vi "Read Configuration.vi"(8 "error in":errorcluster, 11 "Ballard MIL-STD 1553 custom device in":T1 format="%.0x") -> (0 "error out":errorcluster, 2 "1553 channels":T2[](array[typedef]), 3 "Ballard MIL-STD 1553 custom device out":T1 format="%.0x")   [LabVIEW 2020, in "Ballard MIL-STD-1553 Scripting.lvlib"]
uses:
  Ballard MIL-STD-1553 Scripting.lvlib
  <vilib>/NI VeriStand/Custom Device API/Custom Device Item Ref.ctl
  Shared/1553 Channel.ctl
  Shared/Address.ctl
  Shared/Message Definition.ctl
  Shared/Message Type.ctl
  Shared/Terminal Endpoint.ctl
  Shared/Parameter Definition.ctl
  <vilib>/NI VeriStand/Custom Device API/Custom Device API.lvlib
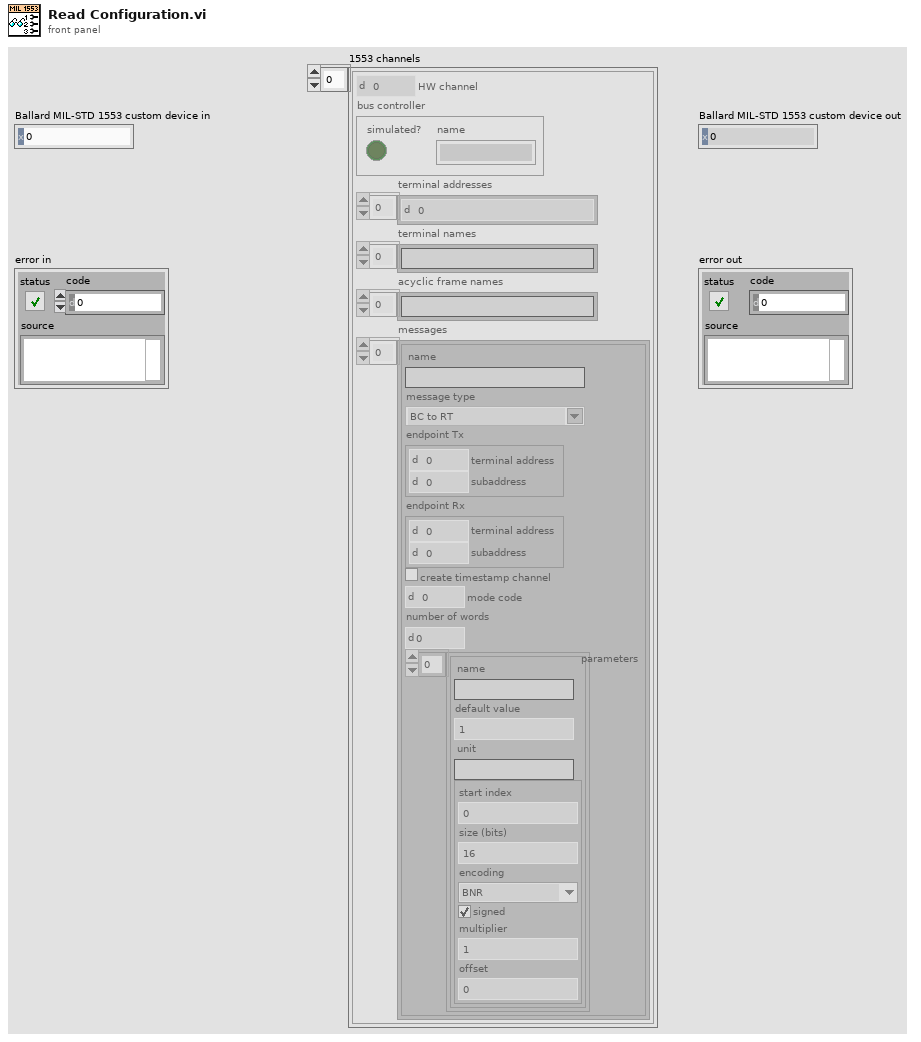
[diagram p1: front panel]
types:
  T1 = typedef "Custom Device API.lvlib/Custom Device Item Ref.ctl" = u64
  T2 = typedef "1553 Channel.ctl" = cluster{"HW channel":u16, "bus controller":cluster{"simulated?":bool, "name":string}, "terminal addresses":T3[], "terminal names":string[], "acyclic frame names":string[], "messages":T4[]}
  T3 = typedef "Address.ctl" = u16
  T4 = typedef "Message Definition.ctl" = cluster{"name":string, "message type":T5, "endpoint Tx":T6, "endpoint Rx":T6, "create timestamp channel":bool, "mode code":u16, "number of words":u16, "parameters":cluster{"name":string, "default value":dbl, "unit":string, "parameter definition":T7}[]}
  T5 = typedef "Message Type.ctl" = string
  T6 = typedef "Terminal Endpoint.ctl" = cluster{"terminal address":T3, "subaddress":T3}
  T7 = typedef "Parameter Definition.ctl" = cluster{"start index":i32, "size (bits)":i32, "encoding":enum16{"BNR", "BCD", "Discrete"}, "signed":bool, "multiplier":dbl, "offset":dbl}
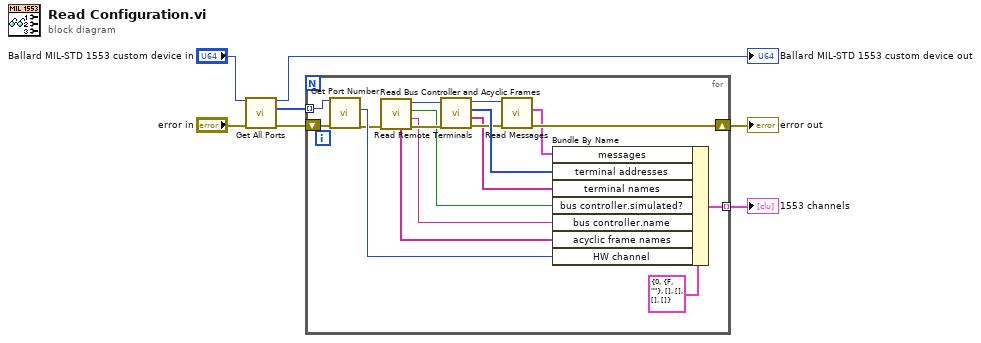
[diagram p0: block diagram]
diagram:
  n1 = call "Get All Ports.vi"("error in"="error in", "Ballard MIL-STD 1553 custom device in"="Ballard MIL-STD 1553 custom device in") -> ("error out"=w4:errorcluster, "ports"=w3:T1[], "Ballard MIL-STD 1553 custom device out"=→"Ballard MIL-STD 1553 custom device out":T1)  [unwired: 7 in]
  n2 = for {
    shift-right: [w16] -> w7
    shift-left: w4 -> [w24]
    tunnel: w3 -> [w23] mode=indexing
    tunnel: [w20] -> w1 mode=indexing
    n3 = call "Get Port Number.vi"("error in"=w24, "port in"=w23) -> ("error out"=w12:errorcluster, "port number"=w21:u16)  [unwired: 6 in, 2 out]
    n4 = call "Read Bus Controller and Acyclic Frames.vi"("error in"=w12) -> ("error out"=w13:errorcluster, "bus controller name"=w9:string, "bus controller found"=w10:bool, "port out"=w8:T1, "acyclic frame names"=w11:string[])  [unwired: 6 in]
    n5 = call "Read Remote Terminals.vi"("error in"=w13, "port in"=w8) -> ("error out"=w17:errorcluster, "terminal names"=w14:string[], "terminals"=w19:T3[], "port out"=w18:T1)  [unwired: 6 in]
    n6 = call "Read Messages.vi"("error in"=w17, "port in"=w18) -> ("error out"=w16:errorcluster, "messages"=w15:T4[])  [unwired: 7 in, 1 out]
    n7 = Bundle By Name(cluster=T2 {"HW channel"=0, "bus controller"={"simulated?"=FALSE, "name"=""}, "terminal addresses"=[], "terminal names"=[], "acyclic frame names"=[], "messages"=[]} ("1553 channel"), "messages"=w15, "terminal addresses"=w19, "terminal names"=w14, "bus controller.simulated?"=w10, "bus controller.name"=w9, "acyclic frame names"=w11, "HW channel"=w21) -> (w20:T2)
  }
  "error out" <- w7
  "1553 channels" <- w1
